vi "PCO_GetConversionFactor.vi"(8 "error in (no error)":errorcluster {"code" format="%x"}, 11 "ph":u64) -> (0 "error out":errorcluster {"code" format="%x"}, 1 "wConvFact":u16, 2 "ErrorMessage":i32 format="%x", 3 "ph out":u64)   [LabVIEW 2020, in "SDK.lvlib" / "ImageSensor.lvlib"]
doc: "<b>Description:</b>\nThis function returns the current conversion factor setting of the image sensor multiplied with the factor 100.\nTo get the current conversion factor in electrons / count the returned value must be divided by 100.\n\n<b>Supported camera type:</b>\nAll cameras\n\n<b>Descriptor dependency:</b>\nNone"
uses:
  ImageSensor.lvlib
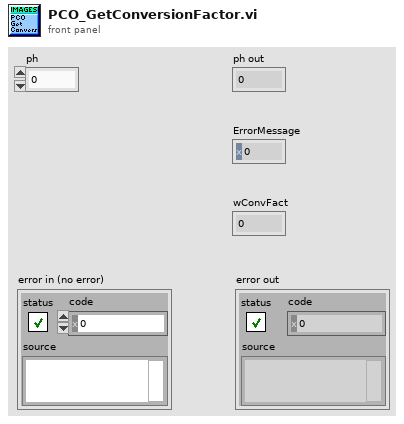
[diagram p1: front panel]
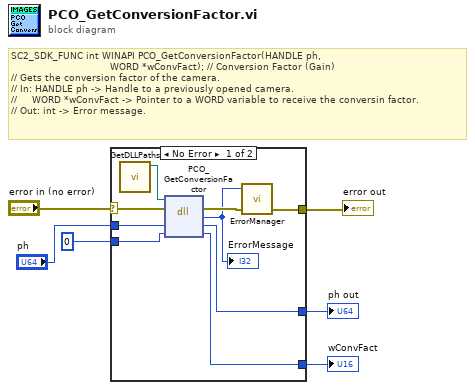
[diagram p0: block diagram]
diagram:
  # "SC2_SDK_FUNC int WINAPI PCO_GetConversionFactor(HANDLE ph,\n                                 WORD *wConvFact); // Conversion Factor (Gain)\n// Gets the conversion factor of the camera.\n// In: HANDLE ph -> Handle to a previously opened camera.\n//     WORD *wConvFact -> Pointer to a WORD variable to receive the conversin factor.\n// Out: int -> Error message."
  n1 = case shown="No Error" "error in (no error)" {
    selector: "error in (no error)" -> [w8 w18]
    tunnel: "ph" -> [w15 w17]
    tunnel: [w14 w17] -> w5
    tunnel: u16 0 ("wConvFact") -> [w13 w16]
    tunnel: [w12 w16] -> w3
    tunnel: [w11 w18] -> w2
    frame No Error {
      n2 = call "GetDLLPaths.vi"() -> ("SC2_Cam_Path"=w7:path)  [unwired: 9 in, 2 out]
      n3 = dll-call lib="?" fn="PCO_GetConversionFactor"(path in=w7, error in=w8, "ph"=w15, "wConvFact"=w13) -> (error out=w10:errorcluster, "return type"=w9:i32, "ph"=w14:u64, "wConvFact"=w12:u16)  [unwired: 1 in, 1 out]
      "ErrorMessage" <- w9
      n4 = call "ErrorManager.vi"("error in (no error)"=w10, "error code"=w9) -> ("error out"=w11:errorcluster)  [unwired: 3 in]
    }
    frame Error {
    }
  }
  "ph out" <- w5
  "wConvFact" <- w3
  "error out" <- w2
